vi "Example Callback.vi"() -> ()   [LabVIEW 2010]
uses:
  C:/tf/play/labview/Tinkerforge.dll
panel:
  in  "stop":bool
  in  "uid":string="63oL6P"
  in  "port":i32=4223
  in  "host":string="localhost"
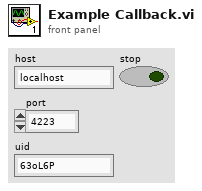
[diagram p1: front panel]
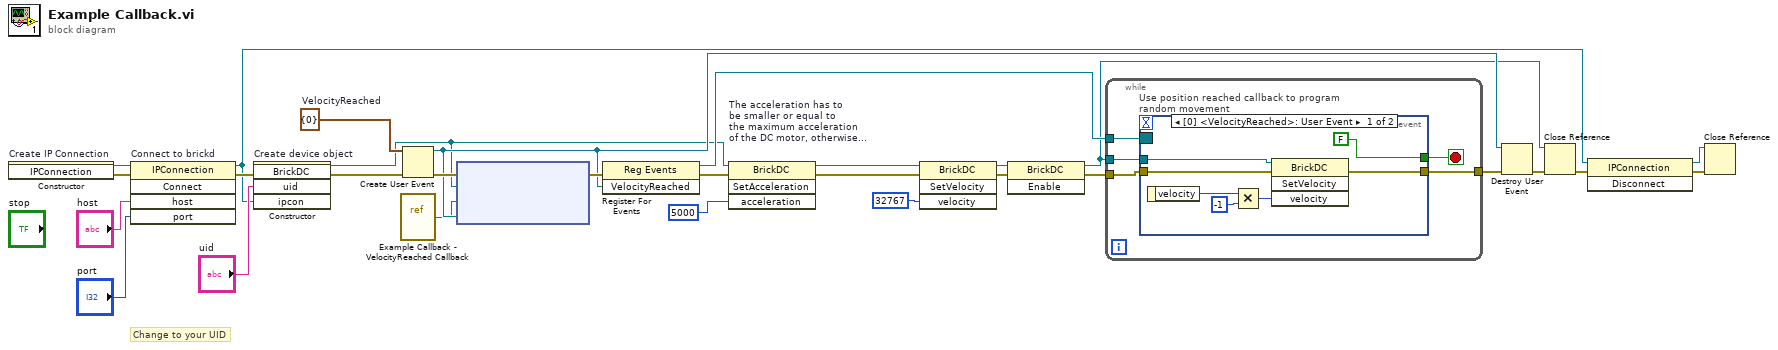
[diagram p0: block diagram]
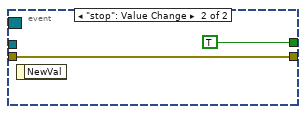
[diagram p2: hidden frame]
diagram:
  w14 = cluster{"velocity":i16} {"velocity"=0}  # VelocityReached
  # "Change to your UID"
  n1 = constructor on="Create IP Connection" class="IPConnection"() -> (reference out=w29:refnum<k24>, error out=w1:errorcluster)  [unwired: 3 in, 1 out]
  n2 = invoke on="Connect to brickd" class="IPConnection" method="Connect"(reference=w29, error in=w1, "host"="host", "port"="port") -> (reference out=w22:refnum<k24>, error out=w25:errorcluster)  [unwired: 1 in, 3 out]
  n3 = constructor on="Create device object" class="BrickDC"(error in=w25, "uid"="uid", "ipcon"=w22) -> (reference out=w12:refnum<k24>, error out=w13:errorcluster)  [unwired: 2 in, 3 out]
  n4 = vi-ref "Example Callback - VelocityReached Callback.vi"() -> ("vi reference"=w7:refnum<vi>)
  n5 = Create User Event(user event datatype=w14, error in=w13) -> (user event=w16:refnum<user-event>, error out=w20:errorcluster)
  n6 = node ("Register Event Callback")(w20, w12, w7, w16) -> (w19:errorcluster)  [unwired: 1 in, 1 out]
  n7 = register-events(error in=w19, w16) -> (reference out=w18:refnum<event-registration>, error out=w11:errorcluster)  [unwired: 1 in]
  n8 = invoke on="The acceleration has to\nbe smaller or equal to\nthe maximum acceleration\nof the DC motor, otherwise\nVelocityReached will be\ncalled too early" class="BrickDC" method="SetAcceleration"(reference=w12, error in=w11, "acceleration"=5000) -> (reference out=w6:refnum<k24>, error out=w5:errorcluster)  [unwired: 1 in, 2 out]
  n9 = invoke class="BrickDC" method="SetVelocity"(reference=w6, error in=w5, "velocity"=i16 32767) -> (reference out=w3:refnum<k24>, error out=w4:errorcluster)  [unwired: 1 in, 2 out]
  n10 = invoke class="BrickDC" method="Enable"(reference=w3, error in=w4) -> (reference out=w9:refnum<k24>, error out=w10:errorcluster)  [unwired: 1 in, 1 out]
  n11 = while {
    tunnel: w18 -> [w34]
    tunnel: [w33] -> w17
    tunnel: w10 -> [w32]
    tunnel: w9 -> [w31]
    stop <- w30 stop-if-true
    n12 = event "Use position reached callback to program random movement" shown="[0] <VelocityReached>: User Event" {
      selector: w34 -> [_ _]
      dyn-events: _ -> [_ _]
      timeout: _ -> [_ _]
      tunnel: [w38 w42] -> w33
      tunnel: w32 -> [w41 w42]
      tunnel: w31 -> [w40 _]
      tunnel: [FALSE TRUE] -> w30
      event User Event {
        n13 = event-data() -> ("velocity"=w37:i16)  [unwired: 1 in]
        n14 = Multiply(x=w37, y=i16 -1) -> (x*y=w36:i16)
        n15 = invoke class="BrickDC" method="SetVelocity"(reference=w40, error in=w41, "velocity"=w36) -> (error out=w38:errorcluster)  [unwired: 1 in, 3 out]
      }
      event "stop": Value Change {
        n16 = event-data() -> ()  [unwired: 1 in, 1 out]
      }
    }
  }
  n17 = Destroy User Event(user event=w16, error in=w17) -> (error out=w15:errorcluster)
  n18 = Close Reference(reference=w9, error in (no error)=w15) -> (error out=w24:errorcluster)
  n19 = invoke class="IPConnection" method="Disconnect"(reference=w22, error in=w24) -> (reference out=w21:refnum<k24>, error out=w23:errorcluster)  [unwired: 1 in, 1 out]
  n20 = Close Reference(reference=w21, error in (no error)=w23) -> ()  [unwired: 1 out]
